vi "LViradon_C.vi"() -> ()   [LabVIEW 2018]
panel:
  in  "IntensityGraph in":refnum<vi>
  in  "IntGraph Refnum":refnum<vi>
  out "Intensity Graph 2":dbl[][](graph)
  out "Intensity Graph":dbl[][](graph)
  in  "2-D Array of Real":dbl[][](array[numeric])
  in  "N_det":dbl=40.0
  in  "N_rot":dbl=40.0
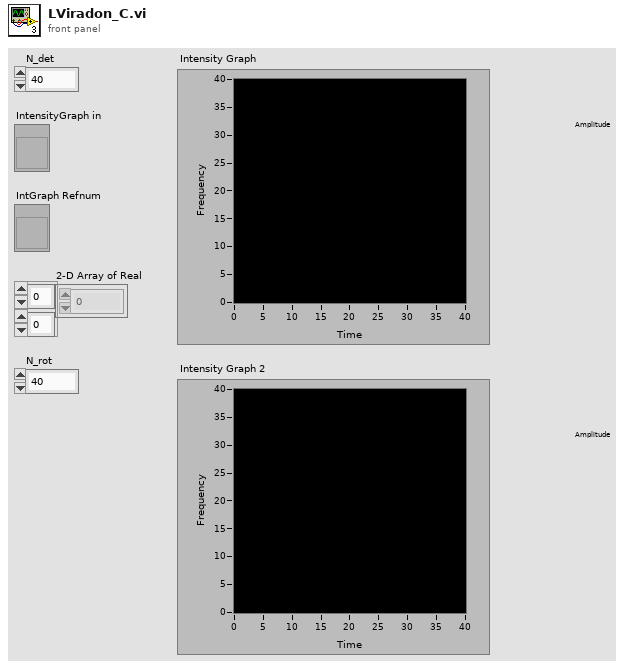
[diagram p1: front panel]
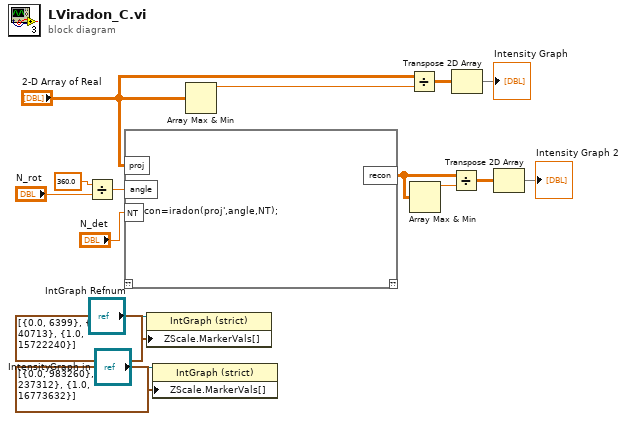
[diagram p0: block diagram]
diagram:
  n1 = Divide(x=360.0, y="N_rot") -> (x/y=w3:dbl)
  n2 = script code="recon=iradon(proj',angle,NT);"("proj"="2-D Array of Real", "angle"=w3, "NT"="N_det") -> ("recon"=w15:dbl[][])  [unwired: 1 in, 1 out]
  n3 = property on="Property Node" class="IntGraph (strict)"(reference="IntGraph Refnum", "ZScale.MarkerVals[]"=cluster{dbl, u32}[] [{0.0, 6399}, {0.5, 40713}, {1.0, 15722240}] ("Z Scale.Marker Values[]")) -> ()  [unwired: 1 in, 2 out]
  n4 = property on="Property Node" class="IntGraph (strict)"(reference="IntensityGraph in", "ZScale.MarkerVals[]"=cluster{dbl, u32}[] [{0.0, 983260}, {0.5, 237312}, {1.0, 16773632}] ("Z Scale.Marker Values[]")) -> ()  [unwired: 1 in, 2 out]
  n5 = Array Max & Min(array="2-D Array of Real") -> (max value=w9:dbl)  [unwired: 3 out]
  n6 = Divide(x="2-D Array of Real", y=w9) -> (x/y=w11:dbl[][])
  n7 = Array Max & Min(array=w15) -> (max value=w16:dbl)  [unwired: 3 out]
  n8 = Divide(x=w15, y=w16) -> (x/y=w13:dbl[][])
  n9 = Transpose 2D Array(2D array=w11) -> (transposed array=→"Intensity Graph":dbl[][])
  n10 = Transpose 2D Array(2D array=w13) -> (transposed array=→"Intensity Graph 2":dbl[][])
